vi "ResumeSong.vi"(8 "error in (no error)":errorcluster, 10 "Message Queues in":T1, 11 "UI Refs in":T2) -> (0 "error out":errorcluster, 2 "Message Queues out":T1, 3 "UI Refs out":T2)   [LabVIEW 2015]
uses:
  Controls & Type Defs/UI Data.ctl
  support/Message Queue/All Message Queues.ctl
  support/Message Queue/Message Cluster.ctl
  support/Message Queue/Enqueue Message (Single).vi
  support/Message Queue/Message Queue.lvlib
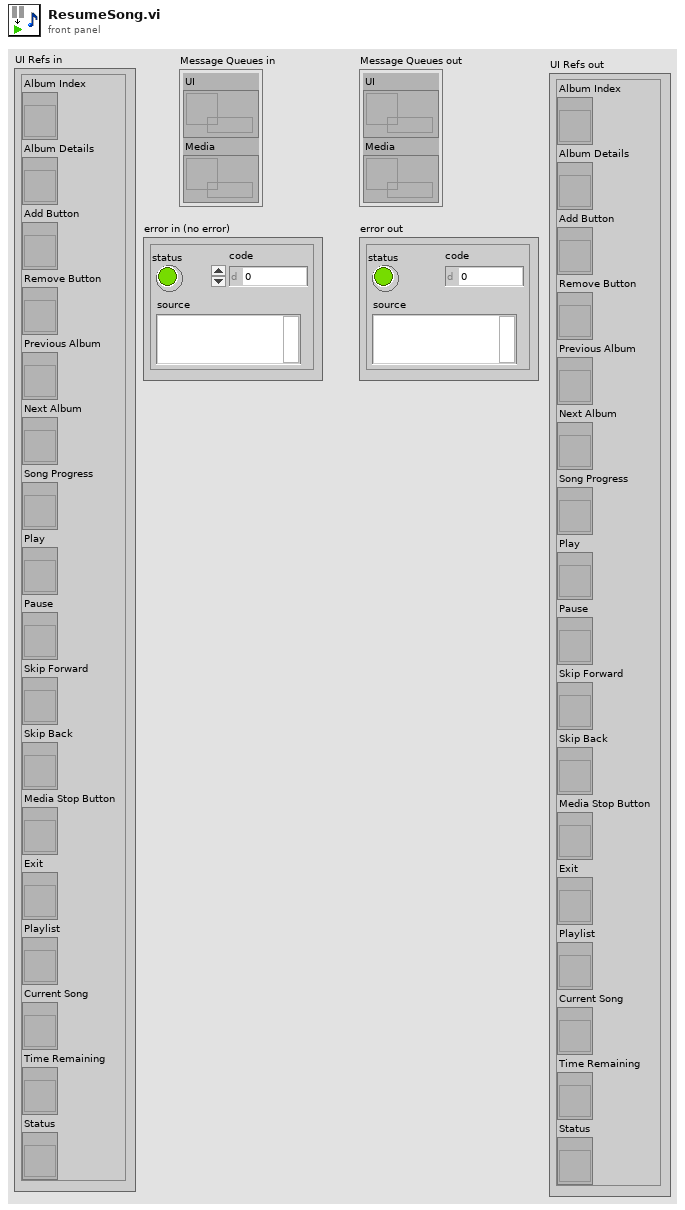
[diagram p1: front panel]
types:
  T1 = typedef "Message Queue.lvlib/All Message Queues.ctl" = cluster{"UI":refnum<queue>, "Media":refnum<queue>}
  T2 = typedef "UI Data.ctl" = cluster{"Album Index":refnum<vi>, "Album Details":refnum<vi>, "Add Button":refnum<vi>, "Remove Button":refnum<vi>, "Previous Album":refnum<vi>, "Next Album":refnum<vi>, "Song Progress":refnum<vi>, "Play":refnum<vi>, "Pause ":refnum<vi>, "Skip Forward":refnum<vi>, "Skip Back":refnum<vi>, "Media Stop Button":refnum<vi>, "Exit":refnum<vi>, "Playlist":refnum<vi>, "Current Song":refnum<vi>, "Time Remaining":refnum<vi>, "Status":refnum<vi>}
  T3 = enum8{"Enabled", "Disabled", "Disabled and Grayed Out"}
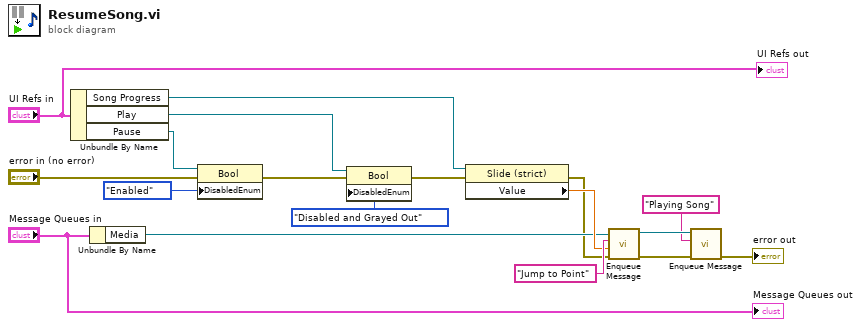
[diagram p0: block diagram]
diagram:
  n1 = Unbundle By Name("UI Refs in") -> ("Song Progress"=w5:refnum<vi>, "Play"=w1:refnum<vi>, "Pause"=w2:refnum<vi>)
  n2 = Unbundle By Name("Message Queues in") -> ("Media"=w14:refnum<queue>)
  n3 = property class="Bool"(reference=w2, "DisabledEnum"=T3."Enabled" ("Disabled")) -> ()  [unwired: 1 in, 2 out]
  n4 = property class="Bool"(reference=w1, "DisabledEnum"=T3."Disabled and Grayed Out" ("Disabled")) -> ()  [unwired: 1 in, 2 out]
  n5 = property class="Slide (strict)"(reference=w5, error in="error in (no error)") -> (error out=w8:errorcluster, "Value"=w15:dbl)  [unwired: 1 out]
  n6 = call-poly "Enqueue Message.vi"("error in (no error)"=w8, "Message Data"=w15, "Message"="Jump to Point", "Message Queue"=w14) -> ("error out"=w10:errorcluster, "dup Message Queue"=w12:refnum<queue>)  [unwired: 6 in]
  n7 = call-poly "Enqueue Message.vi"("error in (no error)"=w10, "Message"="Playing Song", "Message Queue"=w12) -> ("error out"=→"error out":errorcluster)  [unwired: 7 in, 1 out]
  "UI Refs out" <- "UI Refs in"
  "Message Queues out" <- "Message Queues in"
